vi "LEBITplc.BaseInRange.vi"(0 "i ref in":refnum<vi>, 1 "CommandName in":string, 2 "i attribute in":T1, 3 "value":dbl, 5 "error out in":errorcluster) -> (14 "i ref out":refnum<vi>, 15 "CommandName out":string, 18 "In Range?":bool, 19 "error out":errorcluster)   [LabVIEW 2014, in "LEBITplc.lvlib"]
uses:
  LEBITplc.lvlib
  LEBITplc.i attribute.ctl
panel:
  out "i attribute out":T1
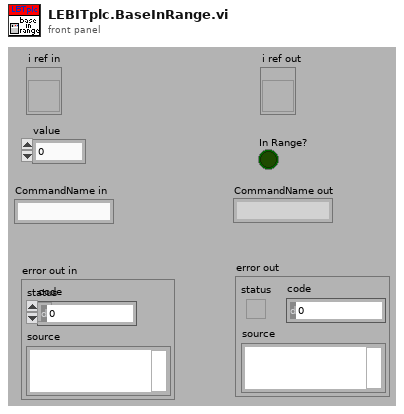
[diagram p1: front panel]
types:
  T1 = typedef "LEBITplc.lvlib/LEBITplc.i attribute.ctl" = cluster{"LLFLocation":string, "SetFileLocation":string, "nickNames":string[], "setValuePLCServiceID":i32[], "GUIServiceID":i32[], "monValuePLC":string[], "SetValueServiceID":i32[], "MonValueServiceID":i32[], "SetValue":dbl[][], "SetValueMin":dbl[], "SetValueMax":dbl[], "SetValueInfoServiceID":i32[], "GUINames":string[], "ListOfBases":string[], "Scale":dbl[], "Offset":dbl[], "setValuePLC":string[], "BaseName":string[], "ScaleServiceID":i32[], "OffsetServiceID":i32[], "AllPLCValues":string[], "CondSpecialArray":string[][], "CondSpecialIndex":i32[], "CondSpecialMonValue":dbl[], "RecentlyChanged":i32[], "SetFileLocationID":i32, "Dependent-Monitors":string[][], "LastLoadedFiles":string[], "IonGuideCalibLocation":string, "Monitor Dependent":string[], "Special":string[], "PLC?":bool[], "Start Date":string, "ListOfBasesServiceID":i32, "SETRA VISA resource":refnum<visa-resource-name>}
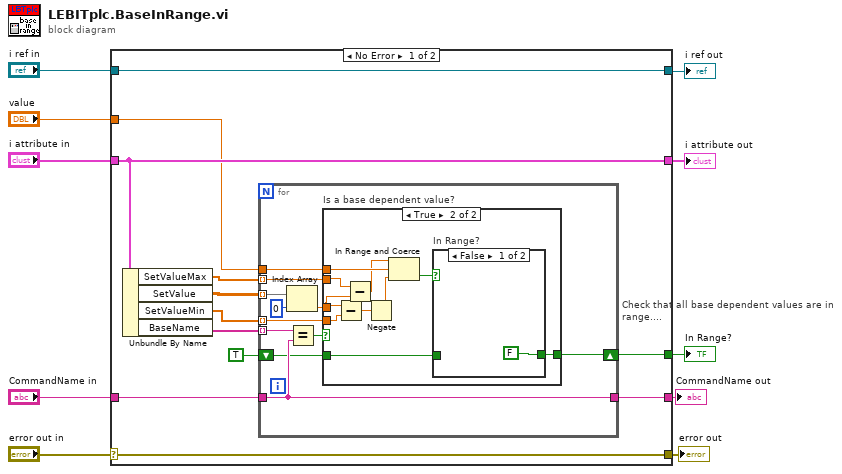
[diagram p0: block diagram]
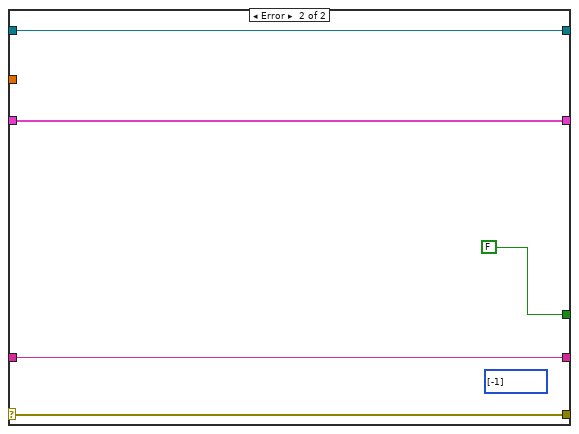
[diagram p4: hidden frame]
diagram:
  n1 = case shown="No Error" "error out in" {
    selector: "error out in" -> [w22 w49]
    tunnel: "i ref in" -> [w21 w51]
    tunnel: "i attribute in" -> [w18 w50]
    tunnel: [w21 w51] -> w6
    tunnel: [w22 w49] -> w7
    tunnel: [w18 w50] -> w5
    tunnel: "CommandName in" -> [w14 w47]
    tunnel: [w12 FALSE] -> w3
    tunnel: [w15 w47] -> w2
    tunnel: "value" -> [w11 _]
    frame No Error {
      n2 = Unbundle By Name(w18) -> ("SetValueMax"=w19:dbl[], "SetValue"=w17:dbl[][], "SetValueMin"=w20:dbl[], "BaseName"=w16:string[])
      n3 = for "Check that all base dependent values are in range...." {
        tunnel: w20 -> [w29] mode=indexing
        tunnel: w19 -> [w30] mode=indexing
        tunnel: w16 -> [w33] mode=indexing
        tunnel: w14 -> [w28]
        tunnel: w11 -> [w31]
        tunnel: w17 -> [w27] mode=indexing
        tunnel: [w28] -> w15
        shift-right: [w23] -> w12
        shift-left: TRUE -> [w24]
        n4 = Index Array(array=w27, index=0) -> (element=w26:dbl)
        n5 = Equal?(x=w33, y=w28) -> (x = y?=w32:bool)
        n6 = case "Is a base dependent value?" shown="True" w32 {
          tunnel: w31 -> [_ w41]
          tunnel: w30 -> [_ w44]
          tunnel: w29 -> [_ w43]
          tunnel: w26 -> [_ w42]
          tunnel: [w34 w39] -> w23
          tunnel: w24 -> [w34 w37]
          frame False {
          }
          frame True {
            n7 = Subtract(x=w42, y=w43) -> (x-y=w38:dbl)
            n8 = Subtract(x=w44, y=w42) -> (x-y=w35:dbl)
            n9 = Negate(x=w38) -> (-x=w36:dbl)
            n10 = In Range and Coerce(upper limit=w35, x=w41, lower limit=w36) -> (In Range?=w40:bool)  [unwired: 1 out]
            n11 = case "In Range?" shown="False" w40 {
              tunnel: [FALSE w46] -> w39
              tunnel: w37 -> [_ w46]
              frame False {
              }
              frame True {
              }
            }
          }
        }
      }
    }
    frame Error {
      (unwired) i32[] [-1]
    }
  }
  "error out" <- w7
  "i attribute out" <- w5
  "i ref out" <- w6
  "In Range?" <- w3
  "CommandName out" <- w2
